vi "showGrid.vi"(6 "Cursor Properties":T1={"Horizontal Line?"=TRUE, "Vertical Line?"=TRUE, "Timestamp"=enum."at BOTTOM", "time format (%H:%M:%S)"="%H:%M:%S", "size"=2, "font"={"Font Name"="Arial", "Size"=16, "Strikeout?"=FALSE, "Italic?"=FALSE, "Underline?"=FALSE, "Outline?"=FALSE, "Shadow"=FALSE, "Bold?"=FALSE}, "alignment(left, top)"={"Horizontal"=enum."center", "Vertical"=enum."center"}, "TextFormat"="%3$s\\n%2$.2f"} {"size" min=1 max=50}, 7 "Picture in":picture, 8 "error in (no error)":errorcluster, 9 "Index":i32, 10 "pixel center":cluster{"horizontal":i16, "vertical":i16}, 11 "QControl_Graph in":refnum<class "QControl_Graph.lvclass">) -> (0 "error out":errorcluster, 3 "QControl_Graph out":refnum<class "QControl_Graph.lvclass">, 5 "Picture out":picture)   [LabVIEW 2017, in "QControl_Graph.lvclass"]
uses:
  QControl_Graph.lvclass
  Applications/National Instruments/LabVIEW 2017 64-bit/vi.lib/QSI/QControls/QControl Classes/WaveformGraph/WaveformGraph.lvclass
  Applications/National Instruments/LabVIEW 2017 64-bit/vi.lib/QSI/QControls/QControl Classes/GraphChart/GraphChart.lvclass
  Cursor Properties.ctl
  Font.ctl
  Alignment.ctl
  Alignment.Horizontal.ctl
  Alignment.Vertical.ctl
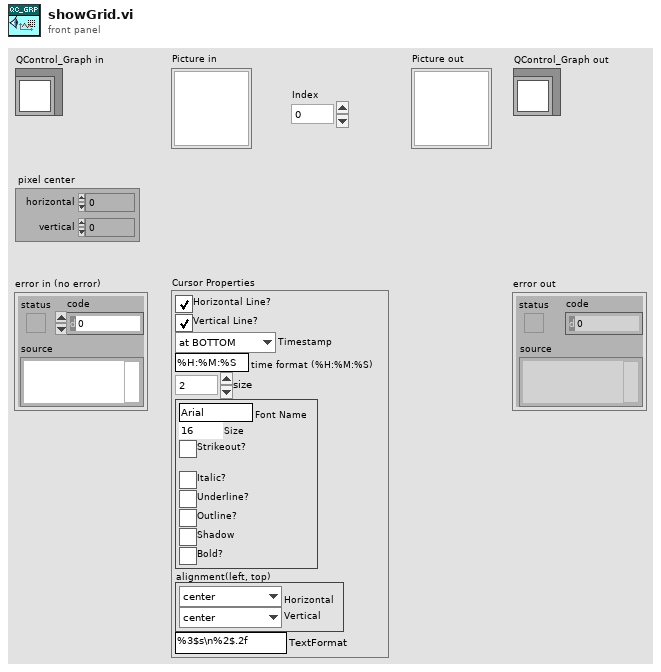
[diagram p1: front panel]
types:
  T1 = typedef "QControl_Graph.lvclass/Cursor Properties.ctl" = cluster{"Horizontal Line?":bool, "Vertical Line?":bool, "Timestamp":enum16{"at TOP", "at BOTTOM", "none"}, "time format (%H:%M:%S)":string, "size":i16, "font":T2, "alignment(left, top)":T3, "TextFormat":string}
  T2 = typedef "QControl_Graph.lvclass/Font.ctl" = cluster{"Font Name":string, "Size":i16, "Strikeout?":bool, "Italic?":bool, "Underline?":bool, "Outline?":bool, "Shadow":bool, "Bold?":bool}
  T3 = typedef "QControl_Graph.lvclass/Alignment.ctl" = cluster{"Horizontal":T4, "Vertical":T5}
  T4 = typedef "QControl_Graph.lvclass/Alignment.Horizontal.ctl" = enum16{"left", "center", "right"}
  T5 = typedef "QControl_Graph.lvclass/Alignment.Vertical.ctl" = enum16{"top", "center", "bottom"}
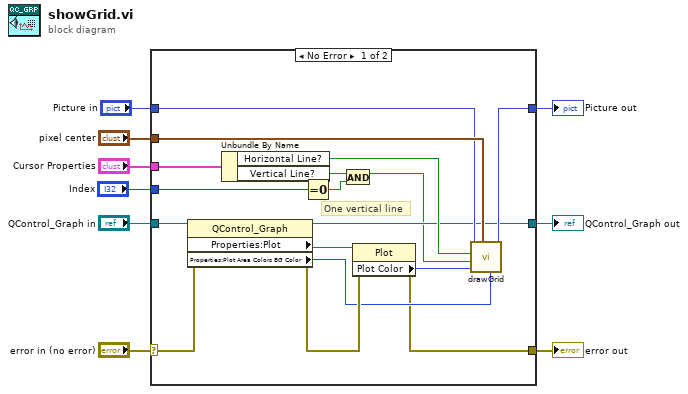
[diagram p0: block diagram]
diagram:
  n1 = case shown="No Error" "error in (no error)" {
    selector: "error in (no error)" -> [w23 w29]
    tunnel: [w13 w29] -> w8
    tunnel: [w14 w28] -> w6
    tunnel: "QControl_Graph in" -> [w26 w28]
    tunnel: "Cursor Properties" -> [w20 _]
    tunnel: "pixel center" -> [w17 _]
    tunnel: "Picture in" -> [w16 w27]
    tunnel: [w15 w27] -> w2
    tunnel: "Index" -> [w12 _]
    frame No Error {
      # "One vertical line"
      n2 = property class="QControl_Graph"(reference=w26, error in=w23) -> (reference out=w14:refnum<class "QControl_Graph.lvclass">, error out=w22:errorcluster, "Properties:Plot"=w25:refnum<vi>, "Properties:Plot Area Colors BG Color"=w21:u32)
      n3 = Unbundle By Name(w20) -> ("Horizontal Line?"=w19:bool, "Vertical Line?"=w18:bool)
      n4 = Equal To 0?(x=w12) -> (x = 0?=w10:bool)
      n5 = And(x=w18, y=w10) -> (x .and. y?=w11:bool)
      n6 = property class="Plot"(reference=w25, error in=w22) -> (error out=w13:errorcluster, "Plot Color"=w24:u32)  [unwired: 1 out]
      n7 = call "drawGrid.vi"("GraphBGK"=w21, "color(black)"=w24, "pixel center"=w17, "Vertical Line?"=w11, "Horizontal Line?"=w19, "picture in"=w16) -> ("picture out"=w15:picture)  [unwired: 5 in]
    }
    frame Error {
    }
  }
  "error out" <- w8
  "QControl_Graph out" <- w6
  "Picture out" <- w2
